vi "Test Storage Global.vi"(7 "Test Label":string, 9 "Clear (F)":bool, 10 "Set (F)":bool, 11 "VI Call Chain":string[](array[string])) -> (1 "Caller ID":string, 2 "Found/Replaced?":bool, 3 "Unique Test ID":string)   [LabVIEW 2013, in "Caraya.lvlib" / "Test Assert Factory.lvclass"]
doc: "Keeps track of VIs that have been registered as tests"
uses:
  Test Assert Factory.lvclass
  Caraya.lvlib
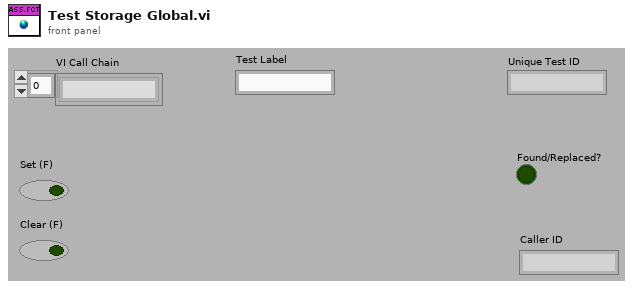
[diagram p1: front panel]
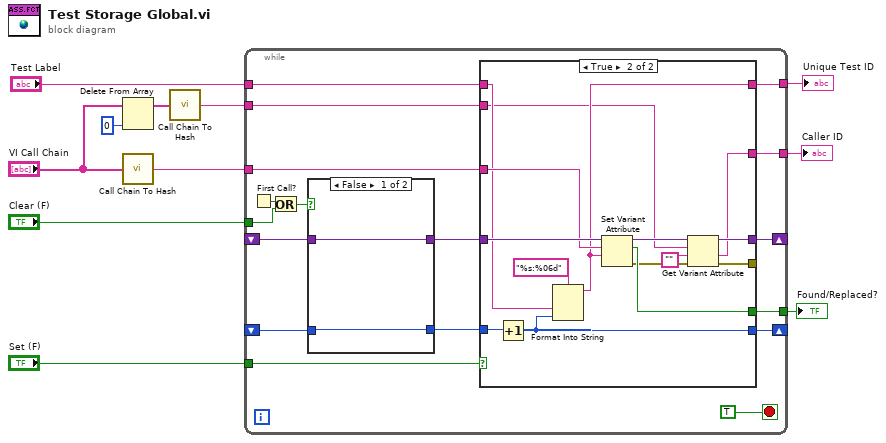
[diagram p0: block diagram]
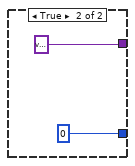
[diagram p2: hidden frame]
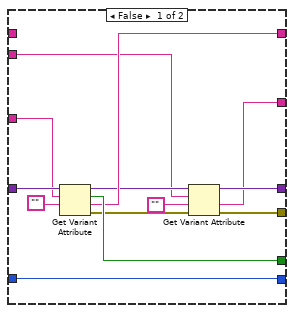
[diagram p3: hidden frame]
diagram:
  n1 = Delete From Array(array="VI Call Chain", index=0) -> (array with subset deleted=w3:string[])  [unwired: 1 in, 1 out]
  n2 = call "Call Chain To Hash.vi"("VI Call Chain"="VI Call Chain") -> ("Key"=w8:string)
  n3 = call "Call Chain To Hash.vi"("VI Call Chain"=w3) -> ("Key"=w2:string)
  n4 = while {
    tunnel: "Set (F)" -> [w27]
    shift-right: [w24] -> _
    shift-left: _ -> [w26]
    tunnel: [w23] -> w10
    tunnel: "Clear (F)" -> [w20]
    tunnel: w8 -> [w19]
    tunnel: [w18] -> w7
    tunnel: "Test Label" -> [w17]
    shift-right: [w15] -> _
    shift-left: _ -> [w14]
    tunnel: w2 -> [w13]
    tunnel: [w12] -> w1
    stop <- TRUE stop-if-true
    n5 = First Call?() -> (First Call?: T/F=w22:bool)
    n6 = Or(x=w22, y=w20) -> (x .or. y?=w21:bool)
    n7 = case shown="False" w21 {
      tunnel: w26 -> [w30 _]
      tunnel: [w30 variant ("variant")] -> w25
      tunnel: [w29 u32 0] -> w16
      tunnel: w14 -> [w29 _]
      frame False {
      }
      frame True {
      }
    }
    n8 = case shown="True" w27 {
      tunnel: w25 -> [w45 w60]
      tunnel: [w39 w51] -> w24
      tunnel: [w44 w59] -> w23
      tunnel: w19 -> [w43 w58]
      tunnel: [w42 w53] -> w18
      tunnel: w17 -> [_ w54]
      tunnel: w16 -> [w41 w57]
      tunnel: [w41 w56] -> w15
      tunnel: w13 -> [w38 w50]
      tunnel: [w35 w48] -> w12
      tunnel: [w34 w47] -> _
      frame False {
        n9 = Get Variant Attribute(Variant=w45, name=w43, default value (empty Variant)="") -> (duplicate Variant=w40:variant, found=w44:bool, value=w42:string, error out=w33:errorcluster)  [unwired: 1 in]
        n10 = Get Variant Attribute(Variant=w40, name=w38, default value (empty Variant)="", error in=w33) -> (duplicate Variant=w39:variant, value=w35:string, error out=w34:errorcluster)  [unwired: 1 out]
      }
      frame True {
        n11 = Increment(x=w57) -> (x+1=w56:u32)
        n12 = Format Into String(format string="%s:%06d", w54, w56) -> (resulting string=w53:string)  [unwired: 2 in, 1 out]
        n13 = Set Variant Attribute(Variant=w60, name=w58, value=w53) -> (Variant out=w52:variant, replaced=w59:bool, error out=w46:errorcluster)  [unwired: 1 in]
        n14 = Get Variant Attribute(Variant=w52, name=w50, default value (empty Variant)="", error in=w46) -> (duplicate Variant=w51:variant, value=w48:string, error out=w47:errorcluster)  [unwired: 1 out]
      }
    }
  }
  "Found/Replaced?" <- w10
  "Unique Test ID" <- w7
  "Caller ID" <- w1
